vi "Set Remote Sense Resistance.vi"(8 "error in (no error)":errorcluster, 10 "Sense Resistance (0)":dbl, 11 "VISA resource name":refnum<visa-resource-name>) -> (0 "error out":errorcluster, 3 "VISA resource name out":refnum<visa-resource-name>)   [LabVIEW 2018, in "XP Power PLS600.lvlib"]
doc: "Sets the Remote Sense Resistance value in Ohms (as opposed to running current through a lead and calculating it)."
uses:
  XP Power PLS600.lvlib
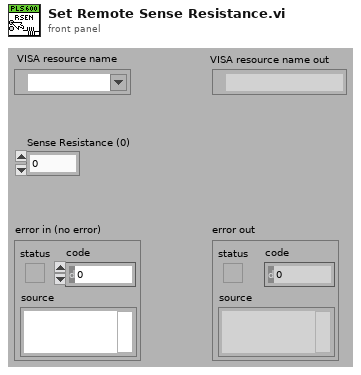
[diagram p1: front panel]
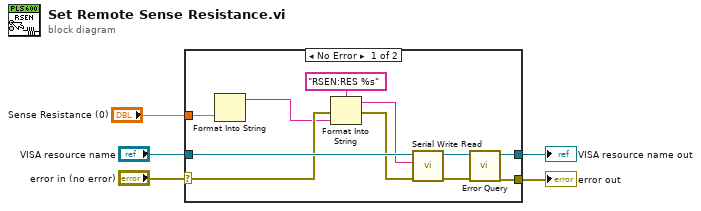
[diagram p0: block diagram]
diagram:
  n1 = case shown="No Error" "error in (no error)" {
    selector: "error in (no error)" -> [w8 w18]
    tunnel: [w16 w17] -> w5
    tunnel: [w15 w18] -> w4
    tunnel: "VISA resource name" -> [w14 w17]
    tunnel: "Sense Resistance (0)" -> [w7 _]
    frame No Error {
      n2 = Format Into String(w7) -> (resulting string=w6:string)  [unwired: 3 in, 1 out]
      n3 = Format Into String(format string="RSEN:RES %s" ("Command to Send"), error in=w8, w6) -> (resulting string=w9:string, error out=w10:errorcluster)  [unwired: 1 in]
      n4 = call "Serial Write Read.vi"("error in (no error)"=w10, "Write Buffer"=w9, "VISA resource name"=w14) -> ("error out"=w12:errorcluster, "VISA resource name out"=w13:refnum<visa-resource-name>)  [unwired: 6 in, 1 out]
      n5 = call "Error Query.vi"("error in (no error)"=w12, "VISA resource name"=w13) -> ("error out"=w15:errorcluster, "VISA resource name out"=w16:refnum<visa-resource-name>)  [unwired: 6 in, 2 out]
    }
    frame Error {
    }
  }
  "VISA resource name out" <- w5
  "error out" <- w4
